vi "jakiPrzedzial.vi"(11 "wejscie":dbl) -> (3 "selector":i16)   [LabVIEW 2020]
doc: "Sprawdzenie czy liczba jest większa, mniejsza czy równa 0.\n\nJeśli wejście > 0, wtedy selector = 1\nJeśli wejście bliskie 0, wtedy selector = 2\nJeśli wejście < 0, wtedy selector = 3"
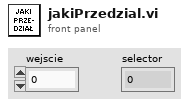
[diagram p1: front panel]
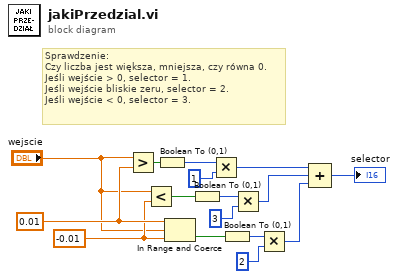
[diagram p0: block diagram]
diagram:
  w16 = 0.01 ("y")
  w15 = -0.01 ("y")
  # "Sprawdzenie:\nCzy liczba jest większa, mniejsza, czy równa 0.\nJeśli wejście > 0, selector = 1.\nJeśli wejście bliskie zeru, selector = 2.\nJeśli wejście < 0, selector = 3."
  n1 = Greater?(x="wejscie", y=w16) -> (0:w1:bool)
  n2 = Less?(x="wejscie", y=w15) -> (x < y?=w2:bool)
  n3 = Boolean To (0,1)(Boolean=w1) -> (0, 1=w3:i16)
  n4 = In Range and Coerce(upper limit=w16, x="wejscie", lower limit=w15) -> (In Range?=w14:bool)  [unwired: 1 out]
  n5 = Boolean To (0,1)(Boolean=w2) -> (0, 1=w4:i16)
  n6 = Multiply(x=w3, y=i16 1) -> (x*y=w8:i16)
  n7 = Boolean To (0,1)(Boolean=w14) -> (0, 1=w5:i16)
  n8 = Multiply(x=w4, y=i16 3) -> (x*y=w9:i16)
  n9 = Multiply(x=w5, y=i16 2) -> (x*y=w10:i16)
  n10 = Compound Arithmetic op=ADD(w8, w9, w10) -> (→"selector":i16)
